vi "Initialise.vi"(8 "EEPROM Size":u16 format="%04x", 9 "EEPROM Base Address":u16 format="%04x", 10 "RAM Size":u16 format="%04x", 11 "RAM Base Address":u16 format="%04x") -> (3 "Memory Map out":refnum<class "Memory Map.lvclass">)   [LabVIEW 2021, in "Memory Map.lvclass"]
uses:
  Memory Map.lvclass
  Memory Range.ctl
  Memory Map.lvclass/Memory Map.ctl
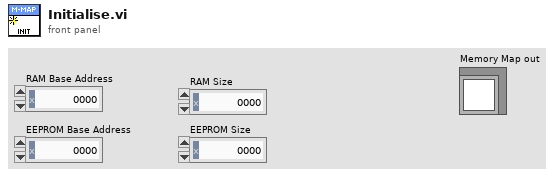
[diagram p1: front panel]
types:
  T1 = typedef "Memory Map.lvclass/Memory Range.ctl" = cluster{"From":u16, "To":u16}
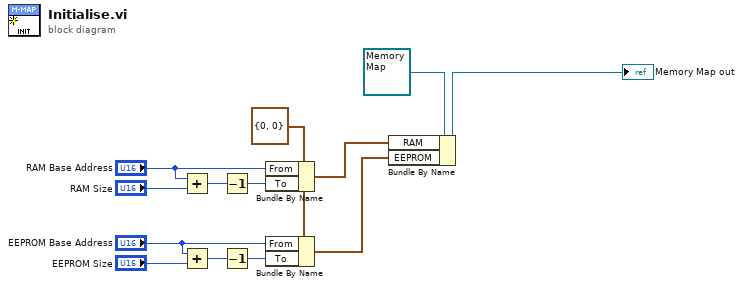
[diagram p0: block diagram]
diagram:
  w10 = T1 {"From"=0, "To"=0} ("RAM")
  n1 = Add(x="RAM Base Address", y="RAM Size") -> (x+y=w7:u16)
  n2 = Add(x="EEPROM Base Address", y="EEPROM Size") -> (x+y=w4:u16)
  n3 = Decrement(x=w7) -> (x-1=w2:u16)
  n4 = Decrement(x=w4) -> (x-1=w1:u16)
  n5 = Bundle By Name(cluster=w10, "From"="RAM Base Address", "To"=w2) -> (w11:T1)
  n6 = Bundle By Name(cluster=w10, "From"="EEPROM Base Address", "To"=w1) -> (w3:T1)
  n7 = Bundle By Name(cluster=refnum<class "Memory Map.lvclass"> refnum ("Memory Map in"), "RAM"=w11, "EEPROM"=w3) -> (→"Memory Map out":refnum<class "Memory Map.lvclass">)
